vi "Result_Test.vi"(8 "error in (no error)":errorcluster caption="entrée d'erreur (pas d'erreur)", 11 "Get_Voltage en entrée":refnum<class "Zigbee_Send_Msg_SwBuildID.lvclass">) -> (0 "error out":errorcluster caption="sortie d'erreur", 3 "Get_Voltage en sortie":refnum<class "Zigbee_Send_Msg_SwBuildID.lvclass">)   [LabVIEW 2020, in "Library Test.lvlib" / "Zigbee_Send_Msg_SwBuildID.lvclass"]
uses:
  Zigbee_Send_Msg_SwBuildID.lvclass
  C:/Users/ngarcin/OneDrive - Altyor/Standard TB/Suite TB45/Class/Test/Zigbee_Send_Msg/Zigbee_Send_Msg.lvclass
  C:/Users/ngarcin/OneDrive - Altyor/Standard TB/Suite TB45/Class/Test/Test (Default)/Test (Default).lvclass
  Commun VI/TypeDef/Variable Printable.ctl
  Zigbee_Send_Msg/Zigbee_Send_Msg.lvclass
  Commun VI/Library Commun.lvlib
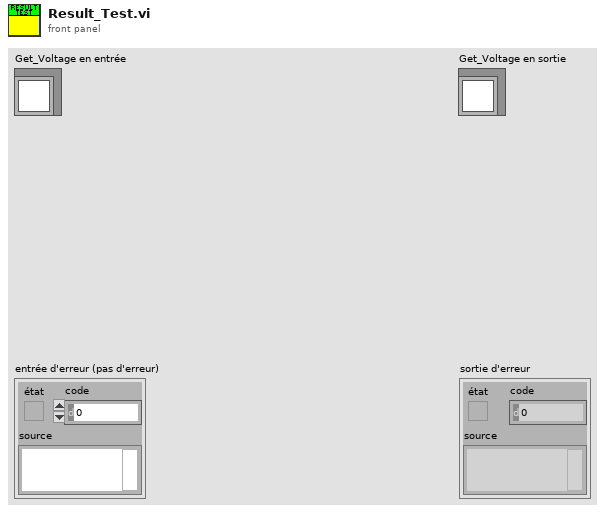
[diagram p1: front panel]
types:
  T1 = typedef "Variable Printable.ctl" = string
  T2 = enum16{"Get Variable", "Get All Variables", "Set Variable", "Delete Variable", "Delete All Variable"}
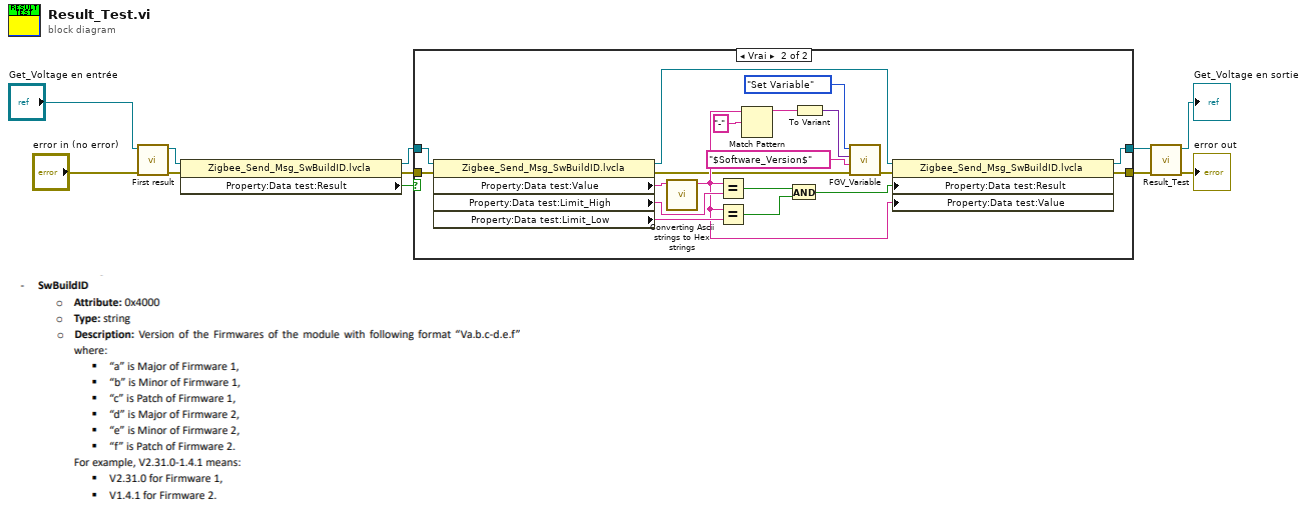
[diagram p0: block diagram]
diagram:
  n1 = call "First result.vi"("entrée d'erreur (pas d'erreur)"="error in (no error)", "Zigbee_Send_Msg en entrée"="Get_Voltage en entrée") -> ("sortie d'erreur"=w3:errorcluster, "Zigbee_Send_Msg en sortie"=w2:refnum<class "Zigbee_Send_Msg_SwBuildID.lvclass">)  [unwired: 7 in, 1 out]
  n2 = property class="Zigbee_Send_Msg_SwBuildID.lvcla"(reference=w2, error in=w3) -> (reference out=w8:refnum<class "Zigbee_Send_Msg_SwBuildID.lvclass">, error out=w9:errorcluster, "Property:Data test:Result"=w10:bool)
  n3 = case shown="Vrai" w10 {
    tunnel: w9 -> [w12 w31]
    tunnel: [w12 w30] -> w11
    tunnel: [w13 w29] -> w6
    tunnel: w8 -> [w13 w28]
    frame False {
    }
    frame True {
      n4 = property class="Zigbee_Send_Msg_SwBuildID.lvcla"(reference=w28, error in=w31) -> (reference out=w32:refnum<class "Zigbee_Send_Msg_SwBuildID.lvclass">, error out=w14:errorcluster, "Property:Data test:Value"=w27:string, "Property:Data test:Limit_High"=w26:string, "Property:Data test:Limit_Low"=w25:string)
      n5 = call "Converting Ascii strings to Hex strings.vi"("result string"=w27) -> ("Chaîne"=w17:string)  [unwired: 10 in]
      n6 = Equal?(x=w17, y=w26) -> (x = y?=w23:bool)
      n7 = Equal?(x=w17, y=w25) -> (x = y?=w24:bool)
      n8 = Match Pattern(string=w17, regular expression="-" ("expression régulière")) -> (before substring=w15:string)  [unwired: 1 in, 3 out]
      n9 = And(x=w23, y=w24) -> (x .and. y?=w22:bool)
      n10 = To Variant(anything=w15) -> (Variant=w20:variant)
      n11 = call "FGV_Variable.vi"("error in (no error)"=w14, "Variable"=T1 "$Software_Version$", "Data In"=w20, "Function"=T2."Set Variable") -> ("error out"=w19:errorcluster)  [unwired: 5 in, 2 out]
      n12 = property class="Zigbee_Send_Msg_SwBuildID.lvcla"(reference=w32, error in=w19, "Property:Data test:Result"=w22, "Property:Data test:Value"=w17) -> (reference out=w29:refnum<class "Zigbee_Send_Msg_SwBuildID.lvclass">, error out=w30:errorcluster)
    }
  }
  n13 = call-parent "Result_Test.vi"("error in (no error)"=w11, "Get_Voltage en entrée"=w6) -> ("error out"=→"error out":errorcluster, "Get_Voltage en sortie"=→"Get_Voltage en sortie":refnum<class "Zigbee_Send_Msg_SwBuildID.lvclass">)  [unwired: 8 in]
